vi "GEOM_SetBinning.vi"(8 "error in (no error)":errorcluster, 10 "Binning In":cluster{"x":u32, "y":u32}={"x"=1, "y"=1} {"y" min=1; "x" min=1}, 11 "binning string":string) -> (0 "error out":errorcluster, 1 "changed":bool, 2 "Binning Out":cluster{"x":u32, "y":u32}={"x"=1, "y"=1} {"y" min=1; "x" min=1})   [LabVIEW 2016]
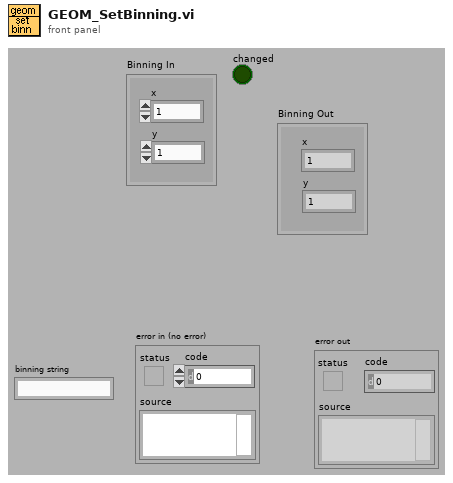
[diagram p1: front panel]
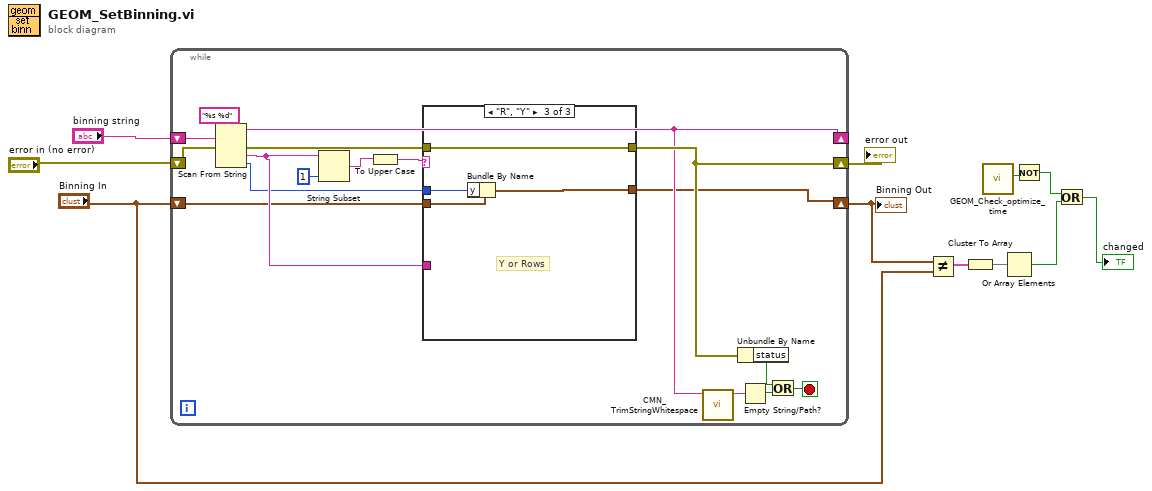
[diagram p0: block diagram]
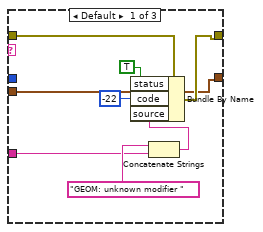
[diagram p2: hidden frame]
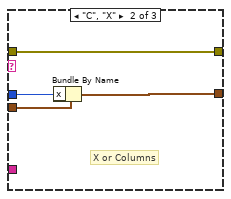
[diagram p3: hidden frame]
diagram:
  n1 = while {
    shift-right: [w20] -> _
    shift-left: "binning string" -> [w28]
    shift-right: [w12] -> w8
    shift-left: "Binning In" -> [w14]
    shift-right: [w22] -> w9
    shift-left: "error in (no error)" -> [w25]
    stop <- w23 stop-if-true
    n2 = Scan From String(format string="%s %d", input string=w28, error in=w25) -> (remaining string=w20:string, error out=w24:errorcluster, output 1=w16:string, output 2=w13:i32)  [unwired: 1 in, 3 out]
    n3 = String Subset(string=w16, length (rest)=1 ("length (rest)")) -> (substring=w17:string)  [unwired: 1 out]
    n4 = To Upper Case(1:w17) -> (0:w18:string)
    n5 = case shown="\"R\", \"Y\"" w18 {
      tunnel: w24 -> [w36 w40 w44]
      tunnel: [w30 w40 w44] -> w22
      tunnel: w16 -> [w32 _ _]
      tunnel: w14 -> [w29 w39 w43]
      tunnel: w13 -> [_ w38 w42]
      tunnel: [w29 w37 w41] -> w12
      frame Default {
        n6 = Concatenate Strings("GEOM: unknown modifier " ("source"), w32) -> (w31:string)
        n7 = Bundle By Name(cluster=w36, "status"=TRUE, "code"=-22, "source"=w31) -> (w30:errorcluster)
      }
      frame "C", "X" {
        # "X or Columns"
        n8 = Bundle By Name(cluster=w39, "x"=w38) -> (w37:cluster{"x":u32, "y":u32})
      }
      frame "R", "Y" {
        # "Y or Rows"
        n9 = Bundle By Name(cluster=w43, "y"=w42) -> (w41:cluster{"x":u32, "y":u32})
      }
    }
    n10 = call "CMN_TrimStringWhitespace.vi"("string"=w20) -> ("trimmed string"=w19:string)  [unwired: 1 in, 8 out]
    n11 = Unbundle By Name(w22) -> ("status"=w21:bool)
    n12 = Empty String/Path?(string/path=w19) -> (empty?=w26:bool)
    n13 = Or(x=w21, y=w26) -> (x .or. y?=w23:bool)
  }
  "error out" <- w9
  "Binning Out" <- w8
  n14 = Not Equal?(x=w8, y="Binning In") -> (x != y?=w6:cluster{"x":bool, "y":bool})
  n15 = Cluster To Array(cluster=w6) -> (array=w5:bool[])
  n16 = call "GEOM_Check_optimize_time.vi"() -> ("optimize"=w4:bool)  [unwired: 11 out]
  n17 = Or Array Elements(Boolean array=w5) -> (logical OR=w2:bool)
  n18 = Not(x=w4) -> (.not. x?=w3:bool)
  n19 = Or(x=w3, y=w2) -> (x .or. y?=→"changed":bool)
